vi "PH_PLH-AccessInformation.constructor.vi"(0 "name":string, 2 "data in":string, 5 "error in(no error)":errorcluster) -> (14 "i ref out":refnum<vi>, 16 "data out":string, 19 "error out":errorcluster)   [LabVIEW 2014, in "PH_PLH-AccessInformation.lvlib"]
doc: "This class is forseen to inspect the PHELIX beamline and to select the mode. Additional several settings can be chosen.\n\nThis class is part of the PHELIX user layer.\n\nauthor: Stefan Götte, GSI\n\nLicense Agreement for this software:\n\nCopyright (C)\nGesellschaft für Schwerionenforschung, GSI\nPlanckstr. 1\n64291 Darmstadt\nGermany\n\nContact: D.Beck@gsi.de \n\nThis program is free software; you can redistribute it and/or modify it under the terms of the \nGNU General Public License as published by the Free Software Foundation; either version 2 of \nthe license, or (at your option) any later version.\n\nThis program is distributed in the hope that it will be useful, but WITHOUT ANY WARRANTY; \nwithout even the implied warranty of MERCHANTABILITY or FITNESS FOR A PARTICULAR PURPOSE. See the GNU General License for more details (http://www.gnu.org).\n\nGesellschaft für Schwerionenforschung, GSI\nPlanckstr. 1, 64291 Darmstadt, Germany\nFor all questions and ideas contact: M.Richter@gsi.de, H.Brand@gsi.de or D.Beck@gsi.de.\nLast update: 16-JUN-2004"
uses:
  PH_PLH-AccessInformation.lvlib
  PH_Basics/PH_Class/PH_Class.lvlib
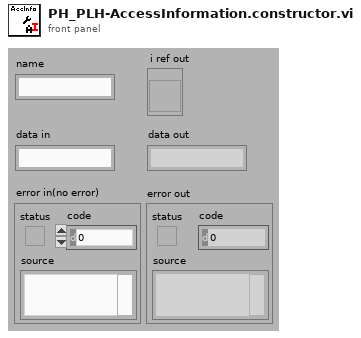
[diagram p1: front panel]
types:
  T1 = enum16{"SetAttribute", "GetAttribute", "CreateAttribute", "DestroyAttribute", "DestroyAllAtributes"}
  T2 = enum16{"no info", "free access", "Searchmode", "Shotmode"}
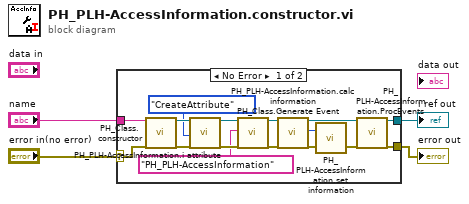
[diagram p0: block diagram]
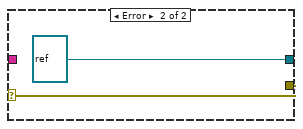
[diagram p2: hidden frame]
diagram:
  n1 = case shown="No Error" "error in(no error)" {
    selector: "error in(no error)" -> [w16 w22]
    tunnel: "name" -> [w17 _]
    tunnel: [w14 w22] -> w3
    tunnel: [w15 refnum<vi> refnum ("i ref out")] -> w2
    frame No Error {
      n2 = call "PH_Class.constructor.vi"("name"=w17, "error in"=w16) -> ("i ref out"=w20:refnum<vi>, "error out"=w19:errorcluster)  [unwired: 15 in, 1 out]
      n3 = call "PH_PLH-AccessInformation.i attribute.vi"("VI Refnum"=w20, "Action"=T1."CreateAttribute", "error in (no error)"=w19) -> ("VI Refnum out"=w6:refnum<vi>, "error out"=w7:errorcluster)  [unwired: 14 in, 1 out]
      n4 = call "PH_Class.Generate Event.vi"("i ref in"=w6, "Class"="PH_PLH-AccessInformation", "error in (no error)"=w7) -> ("i ref out"=w11:refnum<vi>, "error out"=w9:errorcluster)  [unwired: 15 in]
      n5 = call "PH_PLH-AccessInformation.calc information.vi"("i ref in"=w11, "error in"=w9) -> ("i ref out"=w10:refnum<vi>, "Mode"=w12:T2, "error out"=w13:errorcluster)  [unwired: 15 in]
      n6 = call "PH_PLH-AccessInformation.set information.vi"("error in(no error)"=w13, "Mode"=w12) -> ("error out"=w8:errorcluster)
      n7 = call "PH_PLH-AccessInformation.ProcEvents.vi"("i ref in"=w10, "error in (no error)"=w8) -> ("i ref out"=w15:refnum<vi>, "error out"=w14:errorcluster)  [unwired: 16 in]
    }
    frame Error {
    }
  }
  "i ref out" <- w2
  "error out" <- w3
